vi "Motor Controller Datastream (display only).vi"() -> ()   [LabVIEW 2020]
uses:
  ctls/CTRL_Data_Out.ctl
  ctls/CTRL_Cmd.ctl
panel:
  out "Frm err":u32
  out "Chk err":u32
  in  "Set data rate?":bool
  in  "Data rate (Hz)":u8(ring)=14 items=["1", "2", "4", "5", "8", "10", "16", "20", "25", "32", "40", "50", "64", "80", "100", "125", "160", "200", "250", "320", "400", "500", "625", "800", "1000"]
  in  "Stop":bool
  out "Datastream":T1(graph)
  out "Error out":errorcluster
  in  "COM port":refnum<visa-resource-name>
  # "RPM (/min)"
  # "I_m (A)"
  # "Photo (V)"
  # "Duty ()"
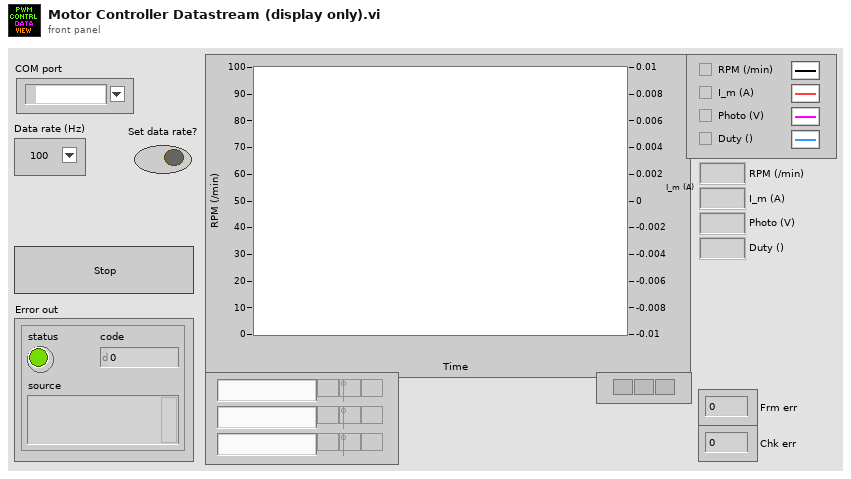
[diagram p1: front panel]
types:
  T1 = cluster{"RPM (/min)":sgl, "I_motor (A)":sgl, "V_photo (V)":sgl, "Duty (-1...1)":sgl}
  T2 = cluster{"RPM (/min)":sgl, "I_motor (A)":sgl, "V_photo (V)":sgl, "Duty (-1...1)":sgl}[]
  T3 = typedef "CTRL_Cmd.ctl" = string
  T4 = typedef "CTRL_Data_Out.ctl" = cluster{"RPM (/min)":sgl, "I_motor (A)":sgl, "V_photo (V)":sgl, "Duty (-1...1)":sgl}
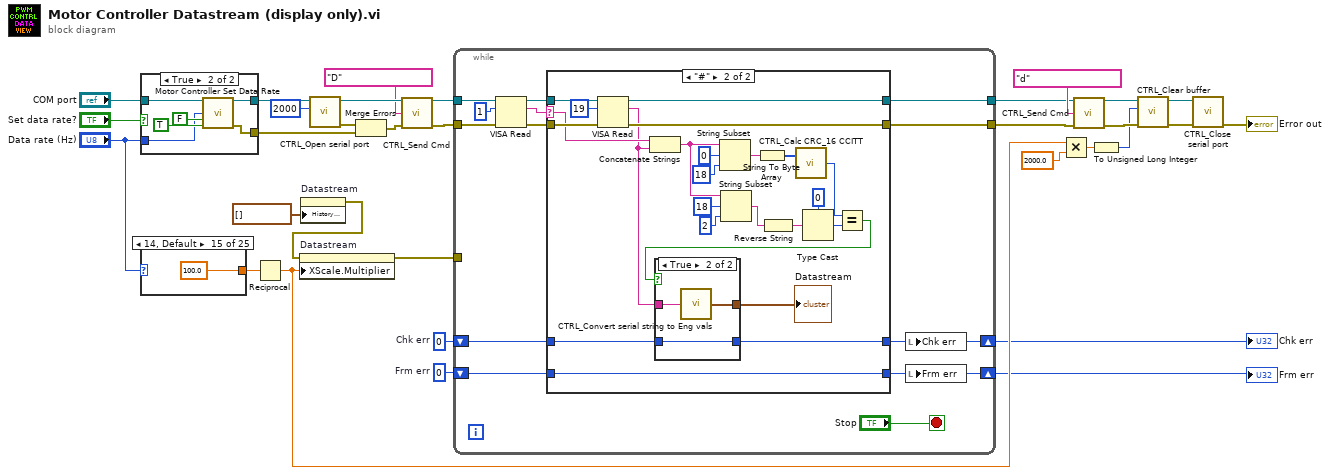
[diagram p0: block diagram]
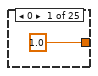
[diagram p2: hidden frame]
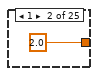
[diagram p3: hidden frame]
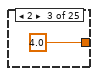
[diagram p4: hidden frame]
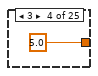
[diagram p5: hidden frame]
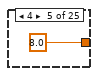
[diagram p6: hidden frame]
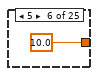
[diagram p7: hidden frame]
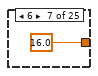
[diagram p8: hidden frame]
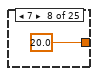
[diagram p9: hidden frame]
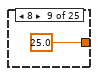
[diagram p10: hidden frame]
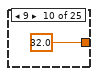
[diagram p11: hidden frame]
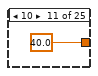
[diagram p12: hidden frame]
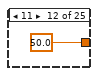
[diagram p13: hidden frame]
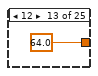
[diagram p14: hidden frame]
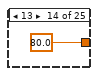
[diagram p15: hidden frame]
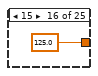
[diagram p16: hidden frame]
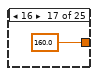
[diagram p17: hidden frame]
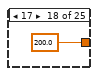
[diagram p18: hidden frame]
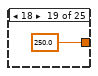
[diagram p19: hidden frame]
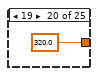
[diagram p20: hidden frame]
diagram:
  w6 = u32 0  # Chk err
  w7 = u32 0  # Frm err
  n1 = case shown="True" "Set data rate?" {
    tunnel: "COM port" -> [w34 w40]
    tunnel: [w34 w39] -> w12
    tunnel: [errorcluster {"status"=FALSE, "code"=0, "source"=""} ("Error out") w38] -> w9
    tunnel: "Data rate (Hz)" -> [_ w35]
    frame False {
    }
    frame True {
      n2 = call "Motor Controller Set Data Rate.vi"("COM port"=w40, "Data rate (Hz)"=w35, "Set as power-on default"=FALSE, "Close port after action"=TRUE) -> ("COM port out"=w39:refnum<visa-resource-name>, "Error out"=w38:errorcluster)  [unwired: 10 in]
    }
  }
  n3 = case shown="14, Default" "Data rate (Hz)" {
    tunnel: [1.0 2.0 4.0 5.0 8.0 10.0 16.0 20.0 25.0 32.0 40.0 50.0 64.0 80.0 100.0 125.0 160.0 200.0 250.0 320.0 400.0 500.0 625.0 800.0 1000.0] -> w2
    frame 0 {
    }
    frame 1 {
    }
    frame 2 {
    }
    frame 3 {
    }
    frame 4 {
    }
    frame 5 {
    }
    frame 6 {
    }
    frame 7 {
    }
    frame 8 {
    }
    frame 9 {
    }
    frame 10 {
    }
    frame 11 {
    }
    frame 12 {
    }
    frame 13 {
    }
    frame 14, Default {
    }
    frame 15 {
    }
    frame 16 {
    }
    frame 17 {
    }
    frame 18 {
    }
    frame 19 {
    }
    frame 20 {
    }
    frame 21 {
    }
    frame 22 {
    }
    frame 23 {
    }
    frame 24 {
    }
  }
  n4 = Reciprocal(x=w2) -> (1/x=w8:dbl)
  n5 = property on="Datastream" class="WFChart (strict)"("History Data"=T2 []) -> (error out=w28:errorcluster)  [unwired: 2 in, 1 out]
  n6 = property on="Datastream" class="WFChart (strict)"(error in=w28, "XScale.Multiplier"=w8) -> (error out=w19:errorcluster)  [unwired: 1 in, 1 out]
  n7 = call "CTRL_Open serial port.vi"("timeout (ms)"=u32 2000, "VISA resource name"=w12) -> ("Error out"=w11:errorcluster, "VISA resource name out"=w16:refnum<visa-resource-name>)  [unwired: 8 in]
  n8 = Merge Errors(w11, w9) -> (w10:errorcluster)
  n9 = call "CTRL_Send Cmd.vi"("Port"=w16, "Cmd"=T3 "D" ("Command"), "Error In"=w10) -> ("Port out"=w17:refnum<visa-resource-name>, "Error Out"=w18:errorcluster)  [unwired: 11 in]
  n10 = while {
    tunnel: w17 -> [w78]
    tunnel: w18 -> [w77]
    tunnel: [w72] -> w25
    tunnel: [w71] -> w26
    tunnel: w19 -> [_]
    shift-right: [w67] -> w3
    shift-left: w7 -> [w70]
    shift-right: [w68] -> w4
    shift-left: w6 -> [w69]
    stop <- "Stop" stop-if-true
    n11 = VISA Read(VISA resource name=w78, byte count=u32 1, error in (no error)=w77) -> (VISA resource name out=w74:refnum<visa-resource-name>, read buffer=w73:string, error out=w75:errorcluster)  [unwired: 1 out]
    n12 = case shown="\"#\"" w73 {
      selector: w73 -> [_ w102]
      tunnel: w75 -> [w83 w106]
      tunnel: w74 -> [w82 w107]
      tunnel: [w83 w104] -> w72
      tunnel: [w82 w103] -> w71
      tunnel: [w81 w87] -> w67
      tunnel: w70 -> [w80 w87]
      tunnel: [w79 w84] -> w68
      tunnel: w69 -> [w79 w86]
      frame Default {
        n13 = Increment(x=w80) -> (x+1=w81:u32)
      }
      frame "#" {
        n14 = VISA Read(VISA resource name=w107, byte count=u32 19, error in (no error)=w106) -> (VISA resource name out=w103:refnum<visa-resource-name>, read buffer=w101:string, error out=w104:errorcluster)  [unwired: 1 out]
        n15 = Concatenate Strings(w102, w101) -> (w89:string)
        n16 = String Subset(string=w89, offset (0)=0, length (rest)=18 ("length (rest)")) -> (substring=w88:string)
        n17 = String Subset(string=w89, offset (0)=18, length (rest)=2 ("length (rest)")) -> (substring=w97:string)
        n18 = String To Byte Array(string=w88) -> (unsigned byte array=w100:u8[])
        n19 = Reverse String(1:w97) -> (0:w95:string)
        n20 = call "CTRL_Calc CRC_16 CCITT.vi"("Data bytes"=w100) -> ("CRC_16-CCITT"=w94:u16)  [unwired: 1 in]
        n21 = Type Cast(type=u16 0 ("length (rest)"), x=w95) -> (*(type *) &x=w93:u16)
        n22 = Equal?(x=w94, y=w93) -> (x = y?=w92:bool)
        n23 = case shown="True" w92 {
          tunnel: w101 -> [_ w113]
          tunnel: [T4 {"RPM (/min)"=nan, "I_motor (A)"=nan, "V_photo (V)"=nan, "Duty (-1...1)"=nan} ("Data") w112] -> w85
          tunnel: [w110 w111] -> w84
          tunnel: w86 -> [w109 w111]
          frame False {
            n24 = Increment(x=w109) -> (x+1=w110:u32)
          }
          frame True {
            n25 = call "CTRL_Convert serial string to Eng vals.vi"("Serial buffer string (excluding FrameChar)"=w113) -> ("Data"=w112:T4)
          }
        }
        "Datastream" <- w85
      }
    }
    n26 = local write "Chk err"(w68) -> ()
    n27 = local write "Frm err"(w67) -> ()
  }
  "Chk err" <- w4
  "Frm err" <- w3
  n28 = Multiply(x=w8, y=2000.0) -> (x*y=w22:dbl)
  n29 = call "CTRL_Send Cmd.vi"("Port"=w26, "Cmd"=T3 "d" ("Command"), "Error In"=w25) -> ("Port out"=w24:refnum<visa-resource-name>, "Error Out"=w23:errorcluster)  [unwired: 11 in]
  n30 = To Unsigned Long Integer(number=w22) -> (unsigned 32bit integer=w20:u32)
  n31 = call "CTRL_Clear buffer.vi"("Error in"=w23, "dt for timeout (ms)"=w20, "VISA resource name in"=w24) -> ("Error out"=w30:errorcluster, "VISA resource name out"=w31:refnum<visa-resource-name>)  [unwired: 3 in]
  n32 = call "CTRL_Close serial port.vi"("Error in"=w30, "VISA resource name"=w31) -> ("Error out"=→"Error out":errorcluster)  [unwired: 9 in]
